vi "Configure Log Mode Sweep.vi"(0 "VISA resource name":refnum<visa-resource-name>, 1 "Source Mode  (0: Voltage)":u16(ring) items=["Voltage", "Current"], 2 "Sweep Points":T1={"Start "=0.1, "Stop "=1.0, "Number of Points (5)"=5}, 3 "Delay (0)":dbl, 4 "Count (1)":i32=1, 5 "error in (no error)":errorcluster, 6 "Fail Abort (T:ON)":bool=TRUE, 7 "Range Type  (1: Best Fixed Range)":u16(ring)=1 items=["Most Sensitive Source Range", "Best Fixed Range", "Present Source Range"], 8 "Dual (F:OFF)":bool, 9 "Buffer Name (defbuffer1)":string="defbuffer1") -> (14 "VISA resource name out":refnum<visa-resource-name>, 19 "error out":errorcluster)   [LabVIEW 2021, in "Keithley 2450.lvlib"]
doc: "Sets up a logarithmic sweep for a set number of measurement points."
uses:
  <instrlib>/Keithley 2450/Keithley 2450.lvlib
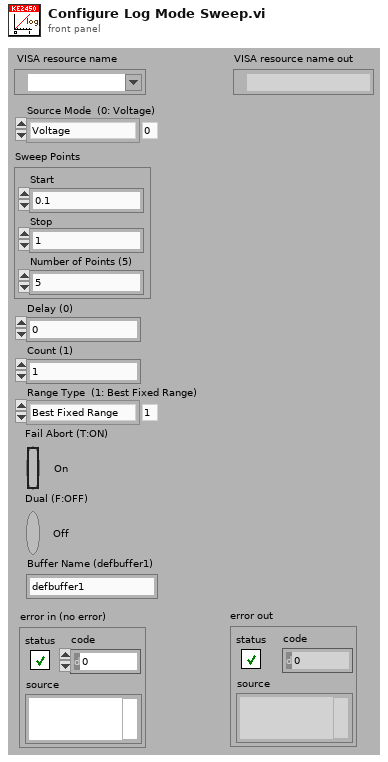
[diagram p1: front panel]
types:
  T1 = cluster{"Start ":dbl, "Stop ":dbl, "Number of Points (5)":u32}
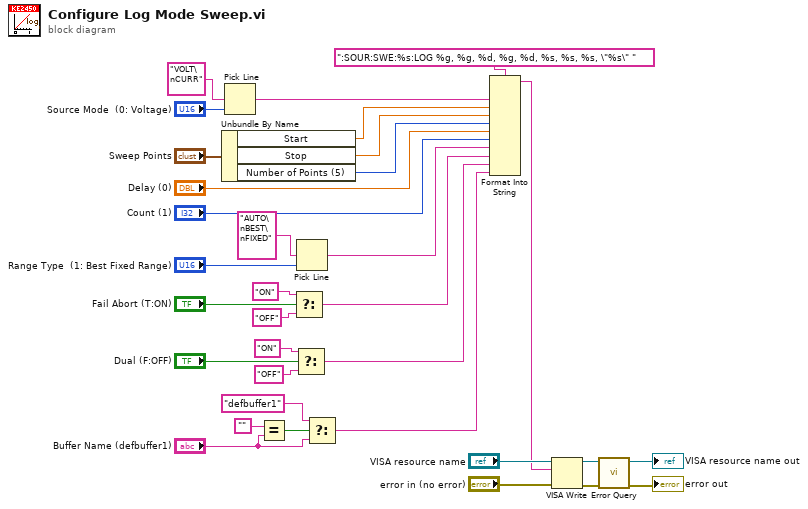
[diagram p0: block diagram]
diagram:
  n1 = Unbundle By Name("Sweep Points") -> ("Start"=w22:dbl, "Stop"=w21:dbl, "Number of Points (5)"=w20:u32)
  n2 = Pick Line(multi-line string="VOLT\nCURR" ("string (\"\")"), line index="Source Mode  (0: Voltage)") -> (output string=w30:string)  [unwired: 1 out]
  n3 = Equal?(x="", y="Buffer Name (defbuffer1)") -> (x = y?=w7:bool)
  n4 = Select(t="ON" ("Buffer Name (defbuffer1)"), s="Fail Abort (T:ON)", f="OFF" ("Buffer Name (defbuffer1)")) -> (s? t:f=w15:string)
  n5 = Select(t="ON" ("Buffer Name (defbuffer1)"), s="Dual (F:OFF)", f="OFF" ("Buffer Name (defbuffer1)")) -> (s? t:f=w9:string)
  n6 = Pick Line(multi-line string="AUTO\nBEST\nFIXED" ("string (\"\")"), line index="Range Type  (1: Best Fixed Range)") -> (output string=w1:string)  [unwired: 1 out]
  n7 = Select(t="defbuffer1", s=w7, f="Buffer Name (defbuffer1)") -> (s? t:f=w5:string)
  n8 = Format Into String(format string=":SOUR:SWE:%s:LOG %g, %g, %d, %g, %d, %s, %s, %s, \"%s\" ", w30, w22, w21, w20, "Delay (0)", "Count (1)", w1, w15, w9, w5) -> (resulting string=w16:string)  [unwired: 2 in, 1 out]
  n9 = VISA Write(VISA resource name="VISA resource name", write buffer=w16, error in (no error)="error in (no error)") -> (VISA resource name out=w27:refnum<visa-resource-name>, error out=w26:errorcluster)  [unwired: 1 out]
  n10 = call <instrlib>:"Error Query.vi"("error in (no error)"=w26, "VISA resource name"=w27) -> ("error out"=→"error out":errorcluster, "VISA resource name out"=→"VISA resource name out":refnum<visa-resource-name>)  [unwired: 8 out]
